vi "test Encode COD-ID.vi"(11 "Test Case In":refnum<class "Passing Tests.lvclass">) -> (0 "error out":errorcluster, 3 "Test Case Out":refnum<class "Passing Tests.lvclass">)   [LabVIEW 2024, in "Passing Tests.lvclass"]
uses:
  Passing Tests.lvclass
  Passing Tests.lvclass/Passing Tests.ctl
  4993e8ee-a06a-463a-9684-69129f64d5ce.vi
  CANopen/CANopen.lvclass
  CANopen/FunctionCode.ctl
  CANopen Master.lvlib
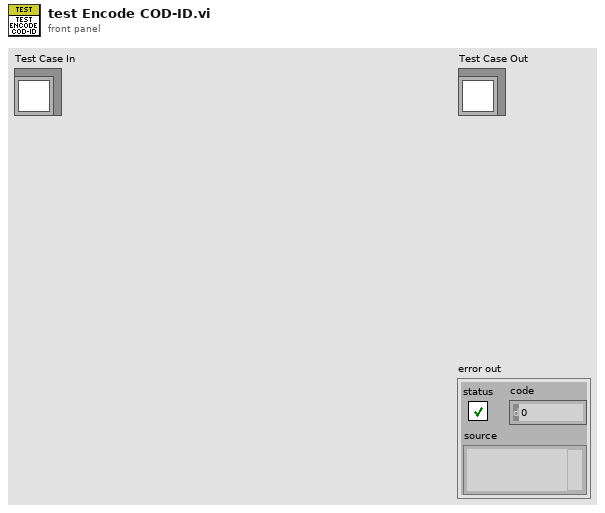
[diagram p1: front panel]
types:
  T1 = typedef "CANopen Master.lvlib/FunctionCode.ctl" = u16
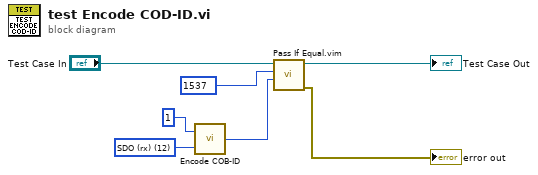
[diagram p0: block diagram]
diagram:
  w4 = T1 12 items=["EMCY"=1, "PDO1 (tx)"=3, "PDO1 (rx)"=4, "PDO2 (tx)"=5, "PDO2 (rx)"=6, "PDO3 (tx)"=7, "PDO3 (rx)"=8, "PDO4 (tx)"=9, "PDO4 (rx)"=10, "SDO (tx)"=11, "SDO (rx)"=12, "NMT error control"=14] ("Function code")
  n1 = call "Encode COB-ID.vi"("Function code"=w4, "Node-ID"=u8 1) -> ("COD-ID"=w1:u32)
  n2 = call "Pass If Equal.vim"("Actual"=w1, "Expected"=u16 1537 ("COD-ID"), "LUnit Test Case In"="Test Case In") -> ("error out"=→"error out":errorcluster, "LUnit Test Case Out"=→"Test Case Out":refnum<class "Passing Tests.lvclass">)  [unwired: 7 in]
